vi "Get Data from String.vi"(8 "error in (no error)":errorcluster, 10 "DataIn":string, 11 "Airmar Data in":refnum<class "Airmar Data.lvclass">) -> (0 "error out":errorcluster, 3 "Airmar Data out":refnum<class "Airmar Data.lvclass">)   [LabVIEW 2015, in "Airmar Data.lvclass"]
uses:
  Airmar Data.lvclass
  Airmar Data.lvclass/Airmar Data.ctl
  Reusable/Data/Write measTime.vi
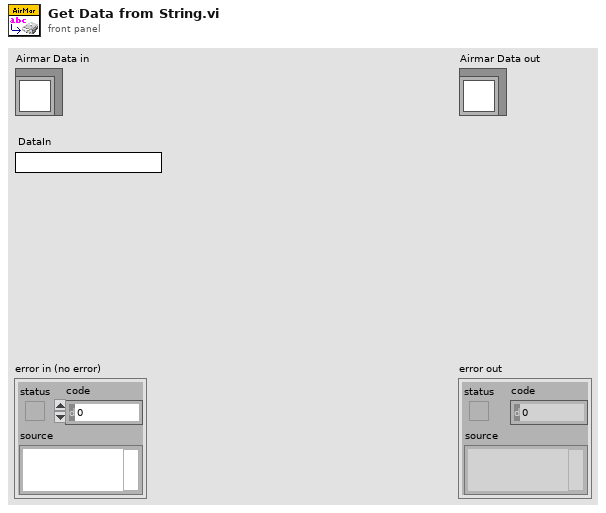
[diagram p1: front panel]
types:
  T1 = enum16{"Fix not available or invalid", "GPS SPS Mode, fix valid", "Differential GPS, SPS Mode, fix valid", "GPS PPS Mode, fix valid", "Real Time Kinematic", "Float RTK", "Estimated (dead reckoning) Mode", "Manual Input Mode", "Simulator Mode"}
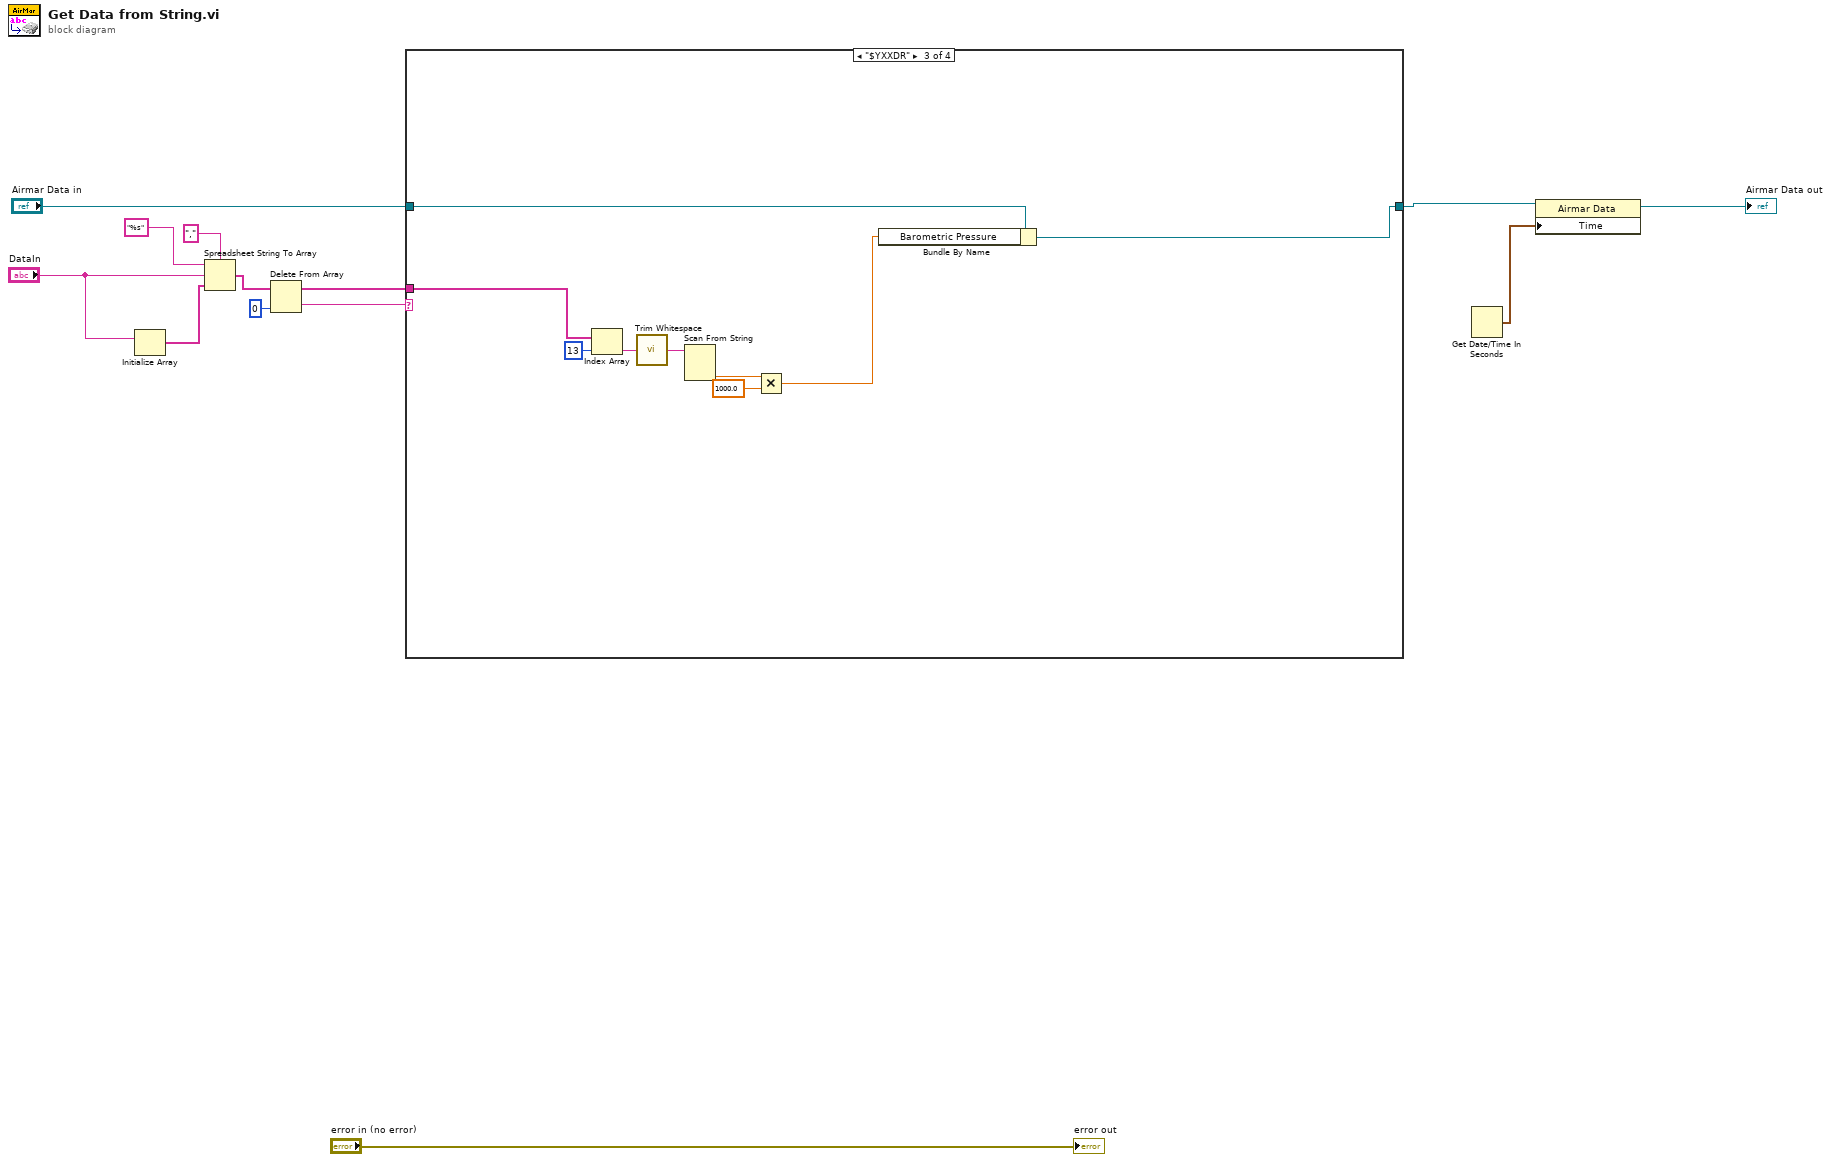
[diagram p0: block diagram]
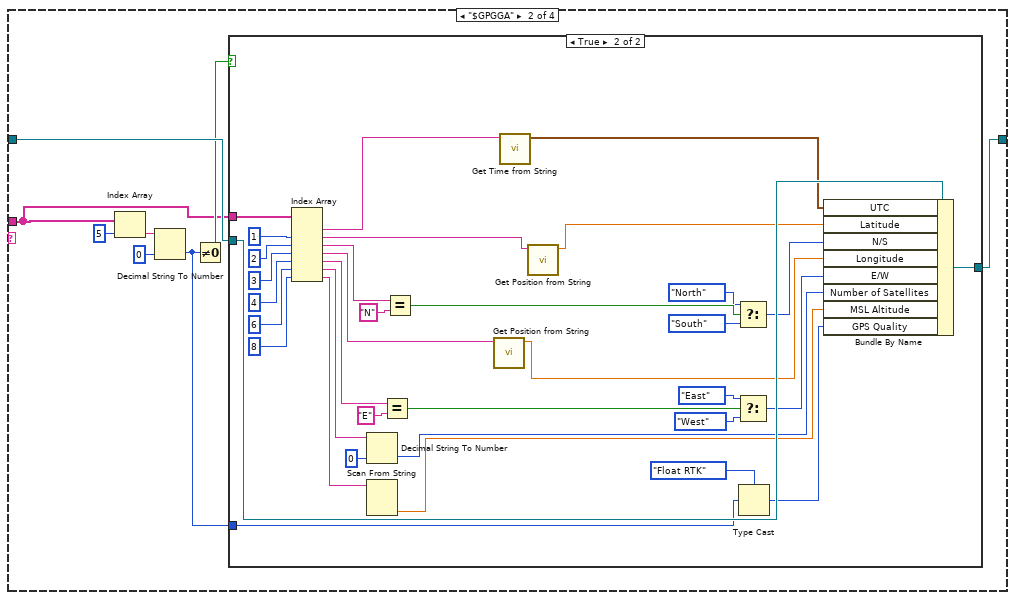
[diagram p3: hidden frame]
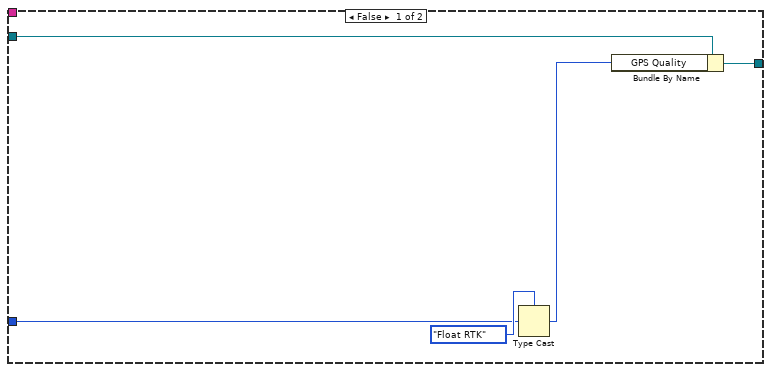
[diagram p4: hidden frame]
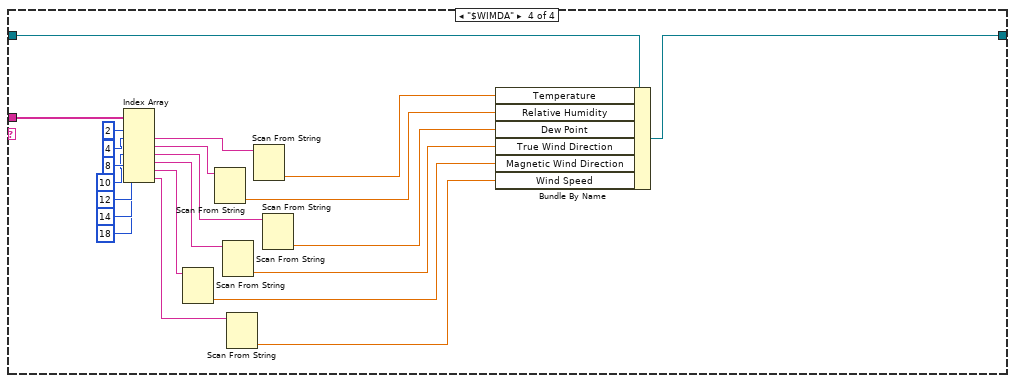
[diagram p5: hidden frame]
diagram:
  n1 = Initialize Array("DataIn") -> (w9:string[])  [unwired: 1 in]
  n2 = Spreadsheet String To Array(delimiter (Tab)=",", format string="%s", spreadsheet string="DataIn", array type (2D Dbl)=w9) -> (array=w8:string[])
  n3 = Delete From Array(array=w8, index=0) -> (deleted portion=w6:string, array with subset deleted=w5:string[])  [unwired: 1 in]
  n4 = case shown="\"$YXXDR\"" w6 {
    tunnel: w5 -> [_ w16 w71 w84]
    tunnel: "Airmar Data in" -> [w14 w22 w66 w93]
    tunnel: [w14 w21 w64 w92] -> w3
    frame "False", Default {
    }
    frame "$GPGGA" {
      n5 = Index Array(array=w16, index=5) -> (element=w19:string)
      n6 = Decimal String To Number(string=w19, default (0L)=u8 0 ("default (0 I32)")) -> (number=w15:u8)  [unwired: 1 in, 1 out]
      n7 = Not Equal To 0?(x=w15) -> (x != 0?=w18:bool)
      n8 = case shown="True" w18 {
        tunnel: w22 -> [w26 w62]
        tunnel: [w27 w61] -> w21
        tunnel: w16 -> [_ w57]
        tunnel: w15 -> [w24 w59]
        frame False {
          n9 = Type Cast(type=T1."Float RTK" ("GGA.GPS Quality"), x=w24) -> (*(type *) &x=w23:T1)
          n10 = Bundle By Name(cluster=w26, "GPS Quality"=w23) -> (w27:refnum<class "Airmar Data.lvclass">)
        }
        frame True {
          n11 = Index Array(array=w57, index #2=1 ("index"), index #3=2 ("index"), index #4=3 ("index"), index #5=4 ("index"), index #6=6 ("index"), index #7=8 ("index")) -> (element #1=w31:string, element #2=w55:string, element #3=w45:string, element #4=w30:string, element #5=w40:string, element #6=w50:string, element #7=w47:string)  [unwired: 1 in]
          n12 = Decimal String To Number(string=w50, default (0L)=u8 0 ("default (0 I32)")) -> (number=w49:u8)  [unwired: 1 in, 1 out]
          n13 = Scan From String(input string=w47) -> (output 1=w46:dbl)  [unwired: 4 in, 3 out]
          n14 = Equal?(x=w40, y="E") -> (x = y?=w38:bool)
          n15 = Equal?(x=w45, y="N") -> (x = y?=w43:bool)
          n16 = call "Get Position from String.vi"("DataIn"=w30) -> ("Numeric"=w29:dbl)  [unwired: 10 in]
          n17 = call "Get Time from String.vi"("DataIn"=w31) -> ("time stamp"=w32:timestamp)  [unwired: 10 in]
          n18 = call "Get Position from String.vi"("DataIn"=w55) -> ("Numeric"=w33:dbl)  [unwired: 10 in]
          n19 = Select(t=enum8{"North", "South"}."North" ("GGA.N/S"), s=w43, f=enum8{"North", "South"}."South" ("GGA.N/S")) -> (s? t:f=w34:enum8{"North", "South"})
          n20 = Select(t=enum8{"East", "West"}."East" ("GGA.E/W"), s=w38, f=enum8{"East", "West"}."West" ("GGA.E/W")) -> (s? t:f=w35:enum8{"East", "West"})
          n21 = Type Cast(type=T1."Float RTK" ("GGA.GPS Quality"), x=w59) -> (*(type *) &x=w58:T1)
          n22 = Bundle By Name(cluster=w62, "UTC"=w32, "Latitude"=w33, "N/S"=w34, "Longitude"=w29, "E/W"=w35, "Number of Satellites"=w49, "MSL Altitude"=w46, "GPS Quality"=w58) -> (w61:refnum<class "Airmar Data.lvclass">)
        }
      }
    }
    frame "$YXXDR" {
      n23 = Index Array(array=w71, index=13) -> (element=w70:string)
      n24 = call <vilib>:"Trim Whitespace.vi"("string"=w70) -> ("trimmed string"=w69:string)  [unwired: 1 in]
      n25 = Scan From String(input string=w69) -> (output 1=w68:dbl)  [unwired: 4 in, 3 out]
      n26 = Multiply(x=w68, y=1000.0) -> (x*y=w65:dbl)
      n27 = Bundle By Name(cluster=w66, "Barometric Pressure"=w65) -> (w64:refnum<class "Airmar Data.lvclass">)
    }
    frame "$WIMDA" {
      n28 = Index Array(array=w84, index #1=2 ("index"), index #2=4 ("index"), index #3=8 ("index"), index #4=10 ("index"), index #5=12 ("index"), index #6=14 ("index"), index #7=18 ("index")) -> (element #2=w83:string, element #3=w82:string, element #4=w81:string, element #5=w80:string, element #6=w75:string, element #7=w73:string)  [unwired: 1 out]
      n29 = Scan From String(input string=w75) -> (output 1=w74:dbl)  [unwired: 4 in, 3 out]
      n30 = Scan From String(input string=w82) -> (output 1=w78:dbl)  [unwired: 4 in, 3 out]
      n31 = Scan From String(input string=w80) -> (output 1=w76:dbl)  [unwired: 4 in, 3 out]
      n32 = Scan From String(input string=w73) -> (output 1=w72:dbl)  [unwired: 4 in, 3 out]
      n33 = Scan From String(input string=w83) -> (output 1=w79:dbl)  [unwired: 4 in, 3 out]
      n34 = Scan From String(input string=w81) -> (output 1=w77:dbl)  [unwired: 4 in, 3 out]
      n35 = Bundle By Name(cluster=w93, "Temperature"=w79, "Relative Humidity"=w78, "Dew Point"=w77, "True Wind Direction"=w76, "Magnetic Wind Direction"=w74, "Wind Speed"=w72) -> (w92:refnum<class "Airmar Data.lvclass">)
    }
  }
  n36 = Get Date/Time In Seconds() -> (seconds since 1Jan1904=w1:timestamp)
  n37 = property class="Airmar Data"(reference=w3, "Time"=w1) -> (reference out=→"Airmar Data out":refnum<class "Airmar Data.lvclass">)  [unwired: 1 in, 1 out]
  "error out" <- "error in (no error)"
